vi "LogisticRegression.vi"(8 "error in":errorcluster) -> (0 "error out":errorcluster, 3 "out":refnum<class "LogisticRegression.lvclass">)   [LabVIEW 2020]
doc: "Logistic Regression (aka logit, MaxEnt) classifier.\n\n In the multiclass case, the training algorithm uses the one-vs-rest (OvR)\n scheme if the 'multi_class' option is set to 'ovr', and uses the\n cross-entropy loss if the 'multi_class' option is set to 'multinomial'.\n (Currently the 'multinomial' option is supported only by the 'lbfgs',\n 'sag', 'saga' and 'newton-cg' solvers.)\n\n This class implements regularized logistic regression using the\n 'liblinear' library, 'newton-cg', 'sag', 'saga' and 'lbfgs' solvers. **Note\n that regularization is applied by default**. It can handle both dense\n and sparse input. Use C-ordered arrays or CSR matrices containing 64-bit\n floats for optimal performance; any other input format will be converted\n (and copied).\n\n The 'newton-cg', 'sag', and 'lbfgs' solvers support only L2 regularization\n with primal formulation, or no regularization. The 'liblinear' solver\n supports both L1 and L2 regularization, with a dual formulation only for\n the L2 penalty. The Elastic-Net regularization is only supported by the\n 'saga' solver.\n\n Read more in the :ref:`User Guide <logistic_regression>`.\n\n Parameters\n ----------\n penalty : {'l1', 'l2', 'elasticnet', 'none'}, default='l2'\n Used to specify the norm used in the penalization. The 'newton-cg',\n 'sag' and 'lbfgs' solvers support only l2 penalties. 'elasticnet' is\n only supported by the 'saga' solver. If 'none' (not supported by the\n liblinear solver), no regularization is applied.\n\n .. versionadded:: 0.19\n l1 penalty with SAGA solver (allowing 'multinomial' + L1)\n\n dual : bool, default=False\n Dual or primal formulation. Dual formulation is only implemented for\n l2 penalty with liblinear solver. Prefer dual=False when\n n_samples > n_features.\n\n tol : float, default=1e-4\n Tolerance for stopping criteria.\n\n C : float, default=1.0\n Inverse of regularization strength; must be a positive float.\n Like in support vector machines, smaller values specify stronger\n regularization.\n\n fit_intercept : bool, default=True\n Specifies if a constant (a.k.a. bias or intercept) should be\n added to the decision function.\n\n intercept_scaling : float, default=1\n Useful only when the solver 'liblinear' is used\n and self.fit_intercept is set to True. In this case, x becomes\n [x, self.intercept_scaling],\n i.e. a \"synthetic\" feature with constant value equal to\n intercept_scaling is appended to the instance vector.\n The intercept becomes ``intercept_scaling * synthetic_feature_weight``.\n\n Note! the synthetic feature weight is subject to l1/l2 regularization\n as all other features.\n To lessen the effect of regularization on synthetic feature weight\n (and therefore on the intercept) intercept_scaling has to be increased.\n\n class_weight : dict or 'balanced', default=None\n Weights associated with classes in the form ``{class_label: weight}``.\n If not given, all classes are supposed to have weight one.\n\n The \"balanced\" mode uses the values of y to automatically adjust\n weights inversely proportional to class frequencies in the input data\n as ``n_samples / (n_classes * np.bincount(y))``.\n\n Note that these weights will be multiplied with sample_weight (passed\n through the fit method) if sample_weight is specified.\n\n .. versionadded:: 0.17\n *class_weight='balanced'*\n\n random_state : int, RandomState instance, default=None\n Used when ``solver`` == 'sag', 'saga' or 'liblinear' to shuffle the\n data. See :term:`Glossary <random_state>` for details.\n\n solver : {'newton-cg', 'lbfgs', 'liblinear', 'sag', 'saga'}, default='lbfgs'\n\n Algorithm to use in the optimization problem.\n\n - For small datasets, 'liblinear' is a good choice, whereas 'sag' and\n 'saga' are faster for large ones.\n - For multiclass problems, only 'newton-cg', 'sag', 'saga' and 'lbfgs'\n handle multinomial loss; 'liblinear' is limited to one-versus-rest\n schemes.\n - 'newton-cg', 'lbfgs', 'sag' and 'saga' handle L2 or no penalty\n - 'liblinear' and 'saga' also handle L1 penalty\n - 'saga' also supports 'elasticnet' penalty\n - 'liblinear' does not support setting ``penalty='none'``\n\n Note that 'sag' and 'saga' fast convergence is only guaranteed on\n features with approximately the same scale. You can\n preprocess the data with a scaler from sklearn.preprocessing.\n\n .. versionadded:: 0.17\n Stochastic Average Gradient descent solver.\n .. versionadded:: 0.19\n SAGA solver.\n .. versionchanged:: 0.22\n The default solver changed from 'liblinear' to 'lbfgs' in 0.22.\n\n max_iter : int, default=100\n Maximum number of iterations taken for the solvers to converge.\n\n multi_class : {'auto', 'ovr', 'multinomial'}, default='auto'\n If the option chosen is 'ovr', then a binary problem is fit for each\n label. For 'multinomial' the loss minimised is the multinomial loss fit\n across the entire probability distribution, *even when the data is\n binary*. 'multinomial' is unavailable when solver='liblinear'.\n 'auto' selects 'ovr' if the data is binary, or if solver='liblinear',\n and otherwise selects 'multinomial'.\n\n .. versionadded:: 0.18\n Stochastic Average Gradient descent solver for 'multinomial' case.\n .. versionchanged:: 0.22\n Default changed from 'ovr' to 'auto' in 0.22.\n\n verbose : int, default=0\n For the liblinear and lbfgs solvers set verbose to any positive\n number for verbosity.\n\n warm_start : bool, default=False\n When set to True, reuse the solution of the previous call to fit as\n initialization, otherwise, just erase the previous solution.\n Useless for liblinear solver. See :term:`the Glossary <warm_start>`.\n\n .. versionadded:: 0.17\n *warm_start* to support *lbfgs*, *newton-cg*, *sag*, *saga* solvers.\n\n n_jobs : int, default=None\n Number of CPU cores used when parallelizing over classes if\n multi_class='ovr'\". This parameter is ignored when the ``solver`` is\n set to 'liblinear' regardless of whether 'multi_class' is specified or\n not. ``None`` means 1 unless in a :obj:`joblib.parallel_backend`\n context. ``-1`` means using all processors.\n See :term:`Glossary <n_jobs>` for more details.\n\n l1_ratio : float, default=None\n The Elastic-Net mixing parameter, with ``0 <= l1_ratio <= 1``. Only\n used if ``penalty='elasticnet'``. Setting ``l1_ratio=0`` is equivalent\n to using ``penalty='l2'``, while setting ``l1_ratio=1`` is equivalent\n to using ``penalty='l1'``. For ``0 < l1_ratio <1``, the penalty is a\n combination of L1 and L2.\n\n Attributes\n ----------\n\n classes_ : ndarray of shape (n_classes, )\n A list of class labels known to the classifier.\n\n coef_ : ndarray of shape (1, n_features) or (n_classes, n_features)\n Coefficient of the features in the decision function.\n\n `coef_` is of shape (1, n_features) when the given problem is binary.\n In particular, when `multi_class='multinomial'`, `coef_` corresponds\n to outcome 1 (True) and `-coef_` corresponds to outcome 0 (False).\n\n intercept_ : ndarray of shape (1,) or (n_classes,)\n Intercept (a.k.a. bias) added to the decision function.\n\n If `fit_intercept` is set to False, the intercept is set to zero.\n `intercept_` is of shape (1,) when the given problem is binary.\n In particular, when `multi_class='multinomial'`, `intercept_`\n corresponds to outcome 1 (True) and `-intercept_` corresponds to\n outcome 0 (False).\n\n n_iter_ : ndarray of shape (n_classes,) or (1, )\n Actual number of iterations for all classes. If binary or multinomial,\n it returns only 1 element. For liblinear solver, only the maximum\n number of iteration across all classes is given.\n\n .. versionchanged:: 0.20\n\n In SciPy <= 1.0.0 the number of lbfgs iterations may exceed\n ``max_iter``. ``n_iter_`` will now report at most ``max_iter``.\n\n See Also\n --------\n SGDClassifier : Incrementally trained logistic regression (when given\n the parameter ``loss=\"log\"``).\n LogisticRegressionCV : Logistic regression with built-in cross validation.\n\n Notes\n -----\n The underlying C implementation uses a random number generator to\n select features when fitting the model. It is thus not uncommon,\n to have slightly different results for the same input data. If\n that happens, try with a smaller tol parameter.\n\n Predict output may not match that of standalone liblinear in certain\n cases. See :ref:`differences from liblinear <liblinear_differences>`\n in the narrative documentation.\n\n References\n ----------\n\n L-BFGS-B -- Software for Large-scale Bound-constrained Optimization\n Ciyou Zhu, Richard Byrd, Jorge Nocedal and Jose Luis Morales.\n http://users.iems.northwestern.edu/~nocedal/lbfgsb.html\n\n LIBLINEAR -- A Library for Large Linear Classification\n https://www.csie.ntu.edu.tw/~cjlin/liblinear/\n\n SAG -- Mark Schmidt, Nicolas Le Roux, and Francis Bach\n Minimizing Finite Sums with the Stochastic Average Gradient\n https://hal.inria.fr/hal-00860051/document\n\n SAGA -- Defazio, A., Bach F. & Lacoste-Julien S. (2014).\n SAGA: A Fast Incremental Gradient Method With Support\n for Non-Strongly Convex Composite Objectives\n https://arxiv.org/abs/1407.0202\n\n Hsiang-Fu Yu, Fang-Lan Huang, Chih-Jen Lin (2011). Dual coordinate descent\n methods for logistic regression and maximum entropy models.\n Machine Learning 85(1-2):41-75.\n https://www.csie.ntu.edu.tw/~cjlin/papers/maxent_dual.pdf\n\n \nAvailable methods:\nGet Attributes\nGet Params\nSet Params"
uses:
  LogisticRegression.lvclass
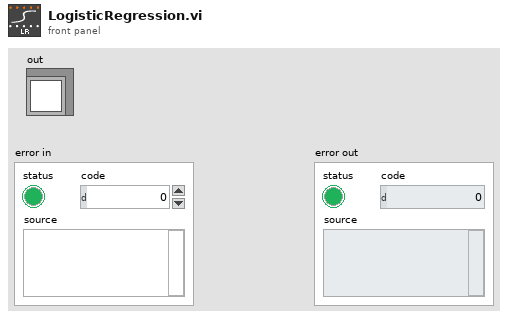
[diagram p1: front panel]
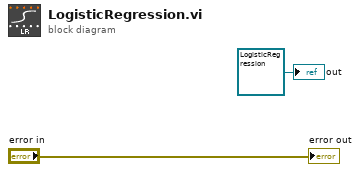
[diagram p0: block diagram]
diagram:
  "out" <- refnum<class "LogisticRegression.lvclass"> refnum ("model")
  "error out" <- "error in"
